vi "Lift.vi"(4 "Set H":bool, 6 "Set L":bool, 7 "Reset":bool, 8 "Lift parameters":T1, 9 "ENC":T2, 10 "Lift Level":dbl, 11 "HG_LIB in":T3) -> (0 "Reset Out":bool, 1 "Lift in  Range":bool, 2 "Lift True":dbl, 3 "Lift Motor":dbl)   [LabVIEW 2020]
uses:
  <vilib>/High Genius/HG_WSI_Tookit/Dependencies/Library/Digital Input and Output/Digital Input and Output.lvclass
panel:
  out "s? t:f":dbl
  out "Lift Level Out":dbl
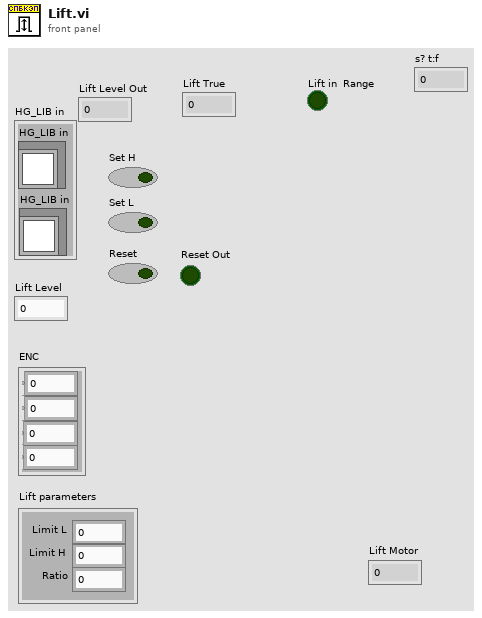
[diagram p1: front panel]
types:
  T1 = cluster{"Limit L":dbl, "Limit H":dbl, "Ratio":dbl}
  T2 = cluster{"ENC Left":i32, "ENC Right":i32, "ENC Back":i32, "ENC Lift":i32}
  T3 = cluster{"HG_LIB in":refnum<class "Digital Input and Output.lvclass">, "HG_LIB in":refnum<class "Digital Input and Output.lvclass">}
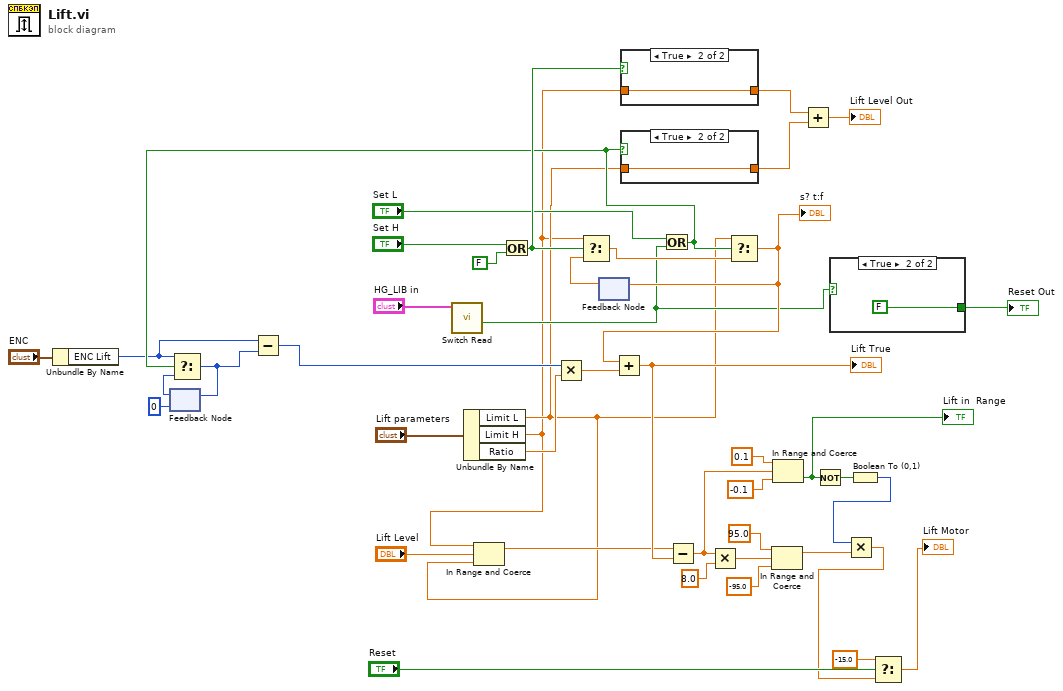
[diagram p0: block diagram]
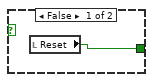
[diagram p2: hidden frame]
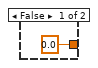
[diagram p3: hidden frame]
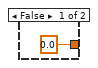
[diagram p4: hidden frame]
diagram:
  n1 = Unbundle By Name("ENC") -> ("ENC Lift"=w19:i32)
  n2 = feedback #1(0) -> (w22:i32)
  n3 = call "Switch Read.vi"("HG_LIB in"="HG_LIB in") -> ("Limit L"=w8:bool)  [unwired: 7 in, 3 out]
  n4 = Unbundle By Name("Lift parameters") -> ("Limit L"=w2:dbl, "Limit H"=w1:dbl, "Ratio"=w16:dbl)
  n5 = In Range and Coerce(upper limit=w1, x="Lift Level", lower limit=w2) -> (coerced(x)=w3:dbl)  [unwired: 1 out]
  n6 = Or(x="Set H", y=FALSE) -> (x .or. y?=w27:bool)
  n7 = feedback #2() -> (w38:dbl)  [unwired: 1 in]
  n8 = Select(t=w1, s=w27, f=w38) -> (s? t:f=w39:dbl)
  n9 = case shown="True" w27 {
    tunnel: [0.0 ("x") w45] -> w24
    tunnel: w1 -> [_ w45]
    frame False {
    }
    frame True {
    }
  }
  n10 = Or(x="Set L", y=w8) -> (x .or. y?=w20:bool)
  n11 = Select(t=w19, s=w20, f=w22) -> (s? t:f=w18:i32)
  n12 = feedback-in #1(w18) -> ()
  n13 = Subtract(x=w19, y=w18) -> (x-y=w17:i32)
  n14 = Multiply(x=w17, y=w16) -> (x*y=w41:dbl)
  n15 = case shown="True" w20 {
    tunnel: [0.0 ("x") w47] -> w25
    tunnel: w2 -> [_ w47]
    frame False {
    }
    frame True {
    }
  }
  n16 = Select(t=w2, s=w20, f=w39) -> (s? t:f=w36:dbl)
  "s? t:f" <- w36
  n17 = feedback-in #2(w36) -> ()
  n18 = Add(x=w36, y=w41) -> (x+y=w15:dbl)
  "Lift True" <- w15
  n19 = Subtract(x=w3, y=w15) -> (x-y=w30:dbl)
  n20 = Multiply(x=w30, y=8.0) -> (x*y=w34:dbl)
  n21 = In Range and Coerce(upper limit=95.0, x=w34, lower limit=-95.0 ("upper limit")) -> (coerced(x)=w31:dbl)  [unwired: 1 out]
  n22 = In Range and Coerce(upper limit=0.1, x=w30, lower limit=-0.1) -> (In Range?=w6:bool)  [unwired: 1 out]
  "Lift in  Range" <- w6
  n23 = Add(x=w24, y=w25) -> (x+y=→"Lift Level Out":dbl)
  n24 = Not(x=w6) -> (.not. x?=w14:bool)
  n25 = case shown="True" w8 {
    tunnel: [w48 FALSE ("Reset Out")] -> w7
    frame False {
      n26 = local read "Reset"() -> (w48:bool)
    }
    frame True {
    }
  }
  "Reset Out" <- w7
  n27 = Boolean To (0,1)(Boolean=w14) -> (0, 1=w13:i16)
  n28 = Multiply(x=w13, y=w31) -> (x*y=w9:dbl)
  n29 = Select(t=-15.0, s="Reset", f=w9) -> (s? t:f=→"Lift Motor":dbl)
